vi "New.vi"(10 "Library Path":path) -> (0 "error in (no error)":errorcluster, 3 "output cluster":refnum<class "lvzstd.lvclass">)   [LabVIEW 2020, in "lvzstd.lvlib" / "lvzstd.lvclass"]
uses:
  lvzstd.lvclass
panel:
  # "Leave library path blank for it to be automatically found"
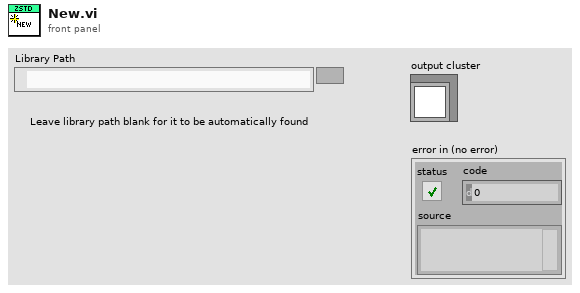
[diagram p1: front panel]
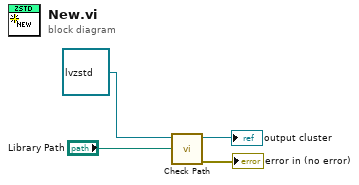
[diagram p0: block diagram]
diagram:
  n1 = call-dynamic "Check Path.vi"("Library Path"="Library Path", "lvzstd in"=refnum<class "lvzstd.lvclass"> refnum ("lvzstd.lvlib:lvzstd.lvclass")) -> ("error in (no error)"=→"error in (no error)":errorcluster, "output lvzstd"=→"output cluster":refnum<class "lvzstd.lvclass">)  [unwired: 8 in]
